vi "SCTLU32toFIFO.vi"(1 "Number":u32, 2 "FifoIn":refnum<k21>) -> (0 "FifoOUT":refnum<k21>)   [LabVIEW 2023]
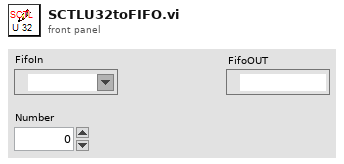
[diagram p1: front panel]
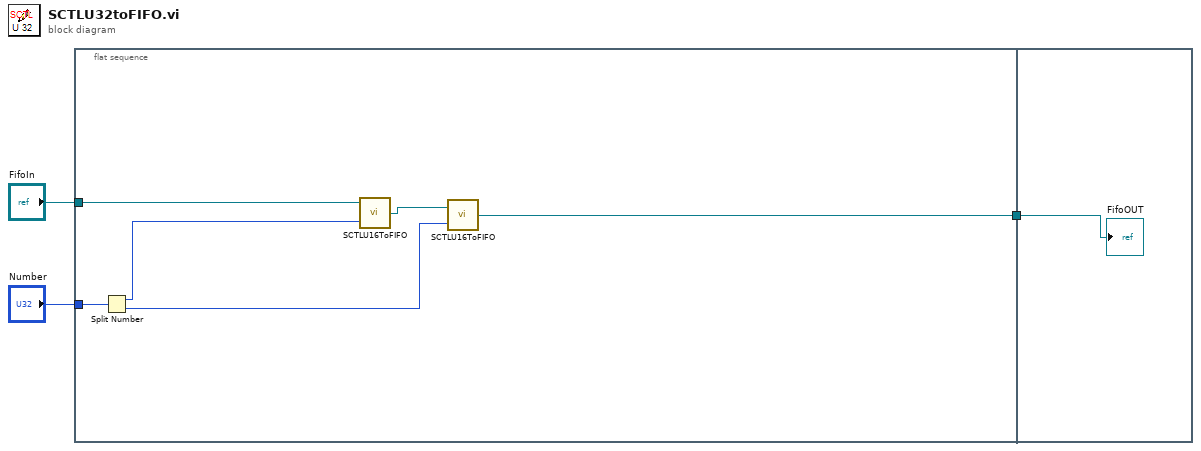
[diagram p0: block diagram]
diagram:
  n1 = flat-sequence {
    tunnel: "Number" -> [w9]
    tunnel: "FifoIn" -> [w8]
    tunnel: [w4] -> w1
    tunnel: w1 -> [w10]
    frame #0 {
      n2 = Split Number(x=w9) -> (hi(x)=w7:u16, lo(x)=w6:u16)
      n3 = call "SCTLU16ToFIFO.vi"("Number"=w7, "FifoIn"=w8) -> ("FifoOUT"=w5:refnum<k21>)
      n4 = call "SCTLU16ToFIFO.vi"("Number"=w6, "FifoIn"=w5) -> ("FifoOUT"=w4:refnum<k21>)
    }
    frame #1 {
      "FifoOUT" <- w10
    }
  }
